vi "Auto Loop 4.vi"(2 "Auto State":u8, 3 "Call Context":T1) -> (1 "SubState 5":T2)   [LabVIEW 2013]
uses:
  typedefs/singleUseSubstate.ctl
  <vilib>/Rock Robotics/WPI/DriverStation/WPI_DriverStationDerivedRobotMode.ctl
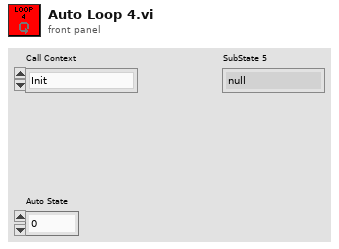
[diagram p1: front panel]
types:
  T1 = typedef "WPI_DriverStationDerivedRobotMode.ctl" = enum16{"Init", "Execute", "Stop"}
  T2 = typedef "singleUseSubstate.ctl" = enum16{"null", "wait", "shift high", "shift low", "extend shooter", "retract shooter", "latch", "unlatch", "end"}
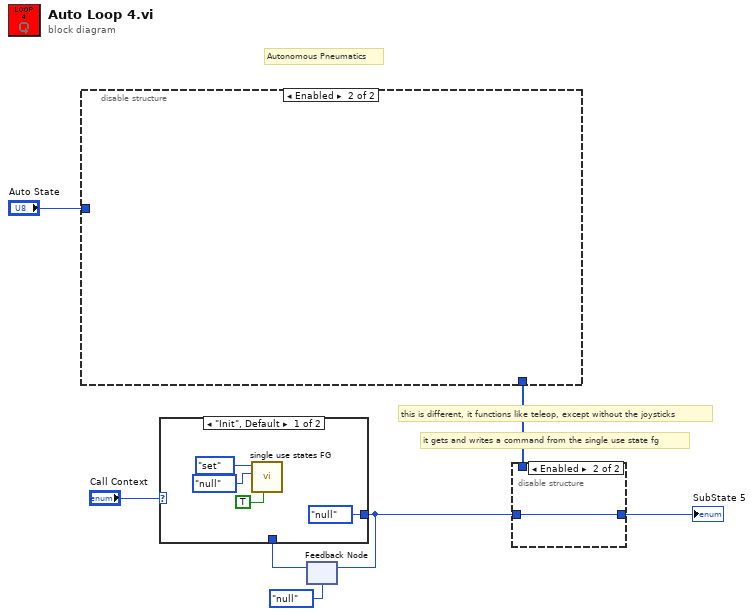
[diagram p0: block diagram]
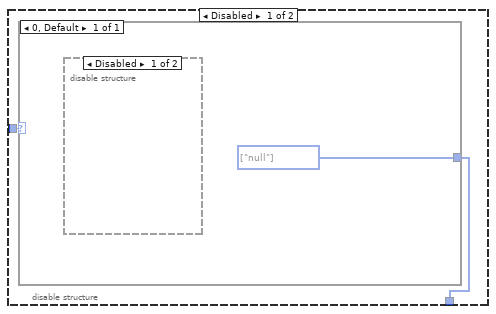
[diagram p2: hidden frame]
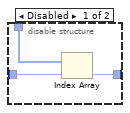
[diagram p4: hidden frame]
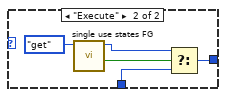
[diagram p5: hidden frame]
diagram:
  # "it gets and writes a command from the single use state fg"
  # "this is different, it functions like teleop, except without the joysticks"
  # "Autonomous Pneumatics"
  n1 = disable-structure shown="Enabled" {
    disable-tunnel: [w9 _] -> w5
    disable-tunnel: "Auto State" -> [w8 _]
    frame Disabled {
      n2 = case shown="0, Default" w8 {
        tunnel: [w10] -> w9
        frame 0, Default {
          w10 = T2[] [enum."null"] items=["null", "wait", "shift high", "shift low", "extend shooter", "retract shooter", "latch", "unlatch", "end"]
          n3 = disable-structure shown="Disabled" {
            frame Disabled {
            }
            frame Enabled {
            }
          }
        }
      }
    }
    frame Enabled {
    }
  }
  n4 = feedback #1(singleUseSubstate."null" ("substate out")) -> (w7:T2)
  n5 = case shown="\"Init\", Default" "Call Context" {
    tunnel: w7 -> [_ w19]
    tunnel: [singleUseSubstate."null" ("substate out") w18] -> w6
    frame "Init", Default {
      n6 = call "single use states FG.vi"("exit in"=TRUE, "substate"=singleUseSubstate."null", "menu (get)"=enum16{"set", "get"}."set") -> ()  [unwired: 5 in, 4 out]
    }
    frame "Execute" {
      n7 = call "single use states FG.vi"("menu (get)"=enum16{"set", "get"}."get") -> ("exit out"=w17:bool, "substate out"=w15:T2)  [unwired: 7 in, 2 out]
      n8 = Select(t=w15, s=w17, f=w19) -> (s? t:f=w18:T2)
    }
  }
  n9 = feedback-in #1(w6) -> ()
  n10 = disable-structure shown="Enabled" {
    disable-tunnel: w6 -> [w22 w23]
    disable-tunnel: w5 -> [w21 _]
    disable-tunnel: [w20 w23] -> w4
    frame Disabled {
      n11 = Index Array(array=w21, index=w22) -> (element=w20:T2)
    }
    frame Enabled {
    }
  }
  "SubState 5" <- w4
